vi "CTR.vi"(0 "System no.":i32=1 min=1 max=4 step=1, 2 "Axes to move":string[](array[string]), 3 "Rel. Target values":dbl[](array[numeric]) format="%.6f", 4 "No.of digits":i16=4, 5 "error in":errorcluster) -> (19 "error out":errorcluster)   [LabVIEW 2020]
doc: "Set relative target value for currently selected control mode. A motion induced by CTR can be interrupted by #24, STP or HLT. Servo must be enabled when commanding CTR. No. of digits is the number of digits after the decimal point in the position value(s) that will be sent.\n\nC-413: Motion commands are not allowed when a wave generator is active or the analog input is used for target generation."
panel:
  # "Set relative target value for currently selected control mode."
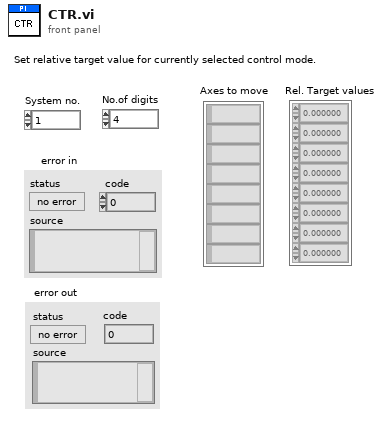
[diagram p1: front panel]
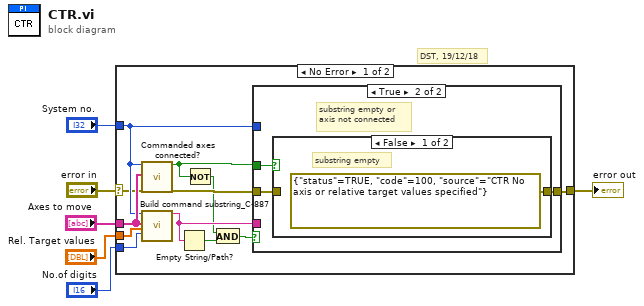
[diagram p0: block diagram]
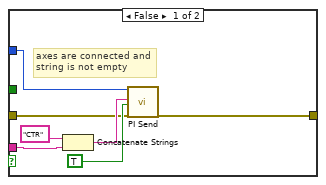
[diagram p2: hidden frame]
diagram:
  # "DST, 19/12/18"
  n1 = case shown="No Error" "error in" {
    selector: "error in" -> [w11 w31]
    tunnel: [w18 w31] -> w6
    tunnel: "Rel. Target values" -> [w17 _]
    tunnel: "No.of digits" -> [w16 _]
    tunnel: "System no." -> [w12 _]
    tunnel: "Axes to move" -> [w14 _]
    frame No Error {
      n2 = call "Commanded axes connected?.vi"("System no."=w12, "Commanded axes"=w14, "error in"=w11) -> ("Controller error"=w8:bool, "error out"=w15:errorcluster)  [unwired: 1 in, 14 out]
      n3 = call "Build command substring_C-887.vi"("System no."=w12, "Affected axes"=w14, "Parameters"=w17, "No. of digits"=w16) -> ("Command substring"=w10:string)  [unwired: 3 in, 12 out]
      n4 = Empty String/Path?(string/path=w10) -> (empty?=w9:bool)
      n5 = Not(x=w8) -> (.not. x?=w7:bool)
      n6 = And(x=w7, y=w9) -> (x .and. y?=w13:bool)
      n7 = case shown="True" w13 {
        tunnel: w10 -> [w19 _]
        tunnel: [w21 w28] -> w18
        tunnel: w15 -> [w22 w26]
        tunnel: w8 -> [_ w27]
        tunnel: w12 -> [w20 _]
        frame False {
          # "axes are connected and \nstring is not empty"
          n8 = Concatenate Strings("CTR", w19) -> (w23:string)
          n9 = call "PI Send.vi"("System no."=w20, "String to send"=w23, "Attach termination char.?"=TRUE ("Attach Linefeed?"), "error in"=w22) -> ("error out"=w21:errorcluster)  [unwired: 2 in, 13 out]
        }
        frame True {
          # "substring empty or \naxis not connected"
          n10 = case shown="False" w27 {
            tunnel: [errorcluster {"status"=TRUE, "code"=100, "source"="CTR No axis or relative target values specified"} ("error out") w30] -> w28
            tunnel: w26 -> [_ w30]
            frame False {
              # "substring empty"
            }
            frame True {
              # "commanded axis \nnot connected"
            }
          }
        }
      }
    }
    frame Error {
    }
  }
  "error out" <- w6
